vi "Read Module Code (Module EEPROM).vi"(8 "error in":errorcluster, 11 "Refnum in":refnum<k20>) -> (0 "error out":errorcluster, 1 "Module ID":u16 format="%x", 2 "Module Code":string, 3 "Refnum out":refnum<k20>)   [LabVIEW 2016, in "SMI.lvlib" / "C Series Module.lvclass"]
uses:
  C Series Module.lvclass
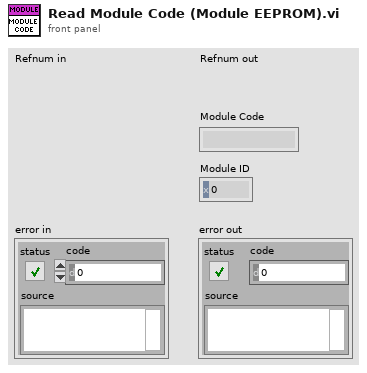
[diagram p1: front panel]
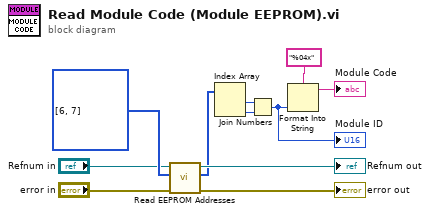
[diagram p0: block diagram]
diagram:
  n1 = call "Read EEPROM Addresses.vi"("error in (no error)"="error in", "Addresses"=u16[] [6, 7], "Refnum in"="Refnum in") -> ("error out"=→"error out":errorcluster, "Data"=w4:u8[], "Refnum out"=→"Refnum out":refnum<k20>)  [unwired: 6 in]
  n2 = Index Array(array=w4) -> (element #1=w2:u8, element #2=w3:u8)  [unwired: 2 in]
  n3 = Join Numbers(hi=w2, lo=w3) -> ((hi.lo)=w1:u16)
  "Module ID" <- w1
  n4 = Format Into String(format string="%04x", w1) -> (resulting string=→"Module Code":string)  [unwired: 2 in, 1 out]
